vi "Set Focus Rects.vi"(8 "error in (no error)":errorcluster, 10 "Focus Rects":T1(array[cluster]), 11 "Scalable Border in":refnum<class "Scalable Border.lvclass">) -> (0 "error out":errorcluster, 3 "Scalable Border out":refnum<class "Scalable Border.lvclass">)   [LabVIEW 2015, in "Scalable Border.lvclass"]
uses:
  Scalable Border.lvclass
  Scalable Border.lvclass/Scalable Border.ctl
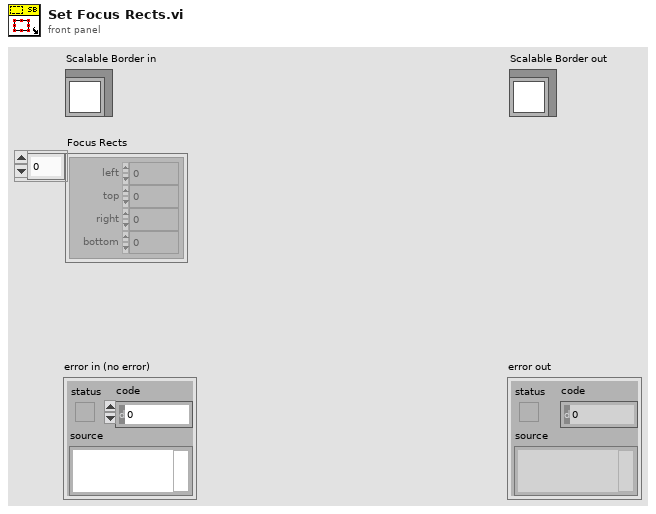
[diagram p1: front panel]
types:
  T1 = cluster{"left":i16, "top":i16, "right":i16, "bottom":i16}[]
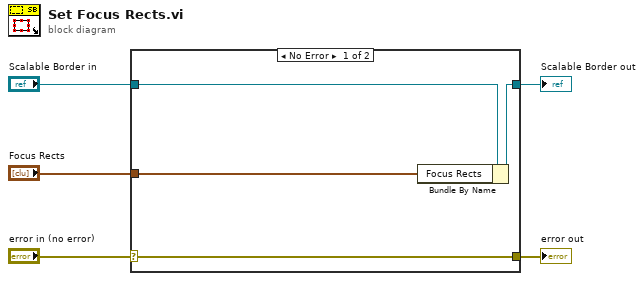
[diagram p0: block diagram]
diagram:
  n1 = case shown="No Error" "error in (no error)" {
    selector: "error in (no error)" -> [w9 w10]
    tunnel: [w9 w10] -> w4
    tunnel: [w7 w11] -> w2
    tunnel: "Scalable Border in" -> [w8 w11]
    tunnel: "Focus Rects" -> [w6 _]
    frame No Error {
      n2 = Bundle By Name(cluster=w8, "Focus Rects"=w6) -> (w7:refnum<class "Scalable Border.lvclass">)
    }
    frame Error {
    }
  }
  "error out" <- w4
  "Scalable Border out" <- w2
